vi "set editor class by value.vi"(8 "error in":errorcluster, 10 "editor":refnum<class "TBM Configuration Node.lvclass">, 11 "configuration in":refnum<class "TBM configuration.lvclass">) -> (0 "error out":errorcluster, 3 "configuration out":refnum<class "TBM configuration.lvclass">)   [LabVIEW 2013, in "PL Framework Configuration Tool.lvlib" / "TBM Configuration Node.lvclass"]
uses:
  TBM Configuration Node.lvclass
  <vilib>/NI/Tag Bus Module Framework/root configuration/TBM configuration.lvclass
  <vilib>/NI/Tag Bus Module Framework/root configuration/set metadata property.vi
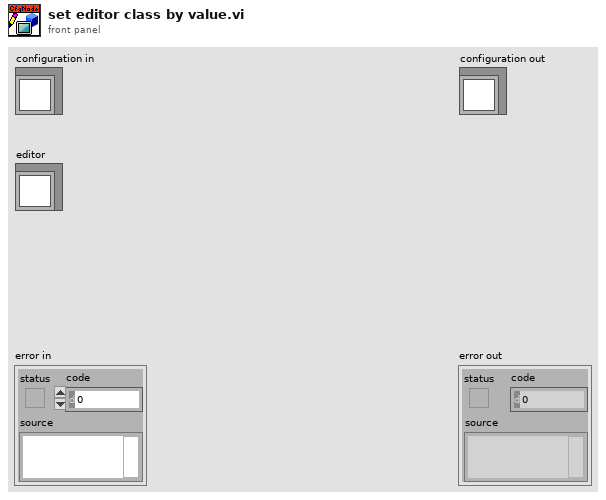
[diagram p1: front panel]
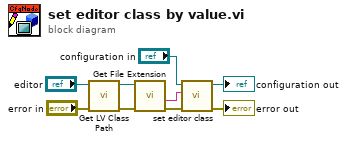
[diagram p0: block diagram]
diagram:
  n1 = call <vilib>:"Get LV Class Path.vi"("error in (no error)"="error in", "object"="editor") -> ("error out"=w9:errorcluster, "class path"=w8:path)  [unwired: 8 in]
  n2 = call <vilib>:"Get File Extension.vi"("error in (no error)"=w9, "file"=w8) -> ("error out"=w2:errorcluster, "filename without extension"=w3:string)  [unwired: 6 in, 2 out]
  n3 = call "set editor class.vi"("error in"=w2, "editor class"=w3, "configuration in"="configuration in") -> ("error out"=→"error out":errorcluster, "configuration out"=→"configuration out":refnum<class "TBM configuration.lvclass">)  [unwired: 7 in]
